vi "Create New Test Case.vi"(8 "error in (no error)":errorcluster, 10 "Path":path, 11 "Application":refnum<vi>) -> (0 "error out":errorcluster)   [LabVIEW 2020]
uses:
  <vilib>/LabVIEW Icon API/lv_icon/classes/Icon/Icon.lvclass
  <vilib>/LabVIEW Icon API/API_Rectangle Dimension.ctl
  <vilib>/LabVIEW Icon API/API_Text.ctl
  <vilib>/LabVIEW Icon API/API_Rectangle Colors.ctl
  <vilib>/Utility/sysdir.llb/System Directory Type.ctl
  <vilib>/Utility/error.llb/Error Cluster From Error Code.vi
  <vilib>/ErrorRing/Error Ring.xnode
  <vilib>/LabVIEW Icon API/LabVIEW Icon API.lvlib
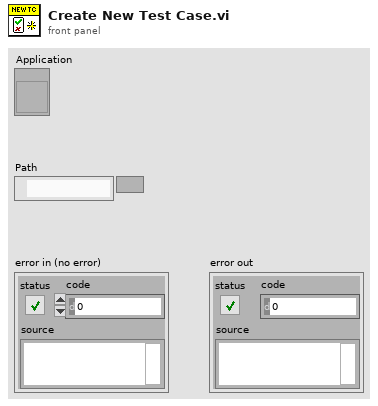
[diagram p1: front panel]
types:
  T1 = typedef "LabVIEW Icon API.lvlib/API_Rectangle Colors.ctl" = cluster{"Border":u32, "Background":u32}
  T2 = typedef "LabVIEW Icon API.lvlib/API_Text.ctl" = cluster{"Line 1 text":string, "Line 2 text":string, "Line 3 text":string, "Line 4 text":string}
  T3 = typedef "LabVIEW Icon API.lvlib/API_Rectangle Dimension.ctl" = cluster{"Width":i16, "Height":i16}
  T4 = typedef "System Directory Type.ctl" = i32
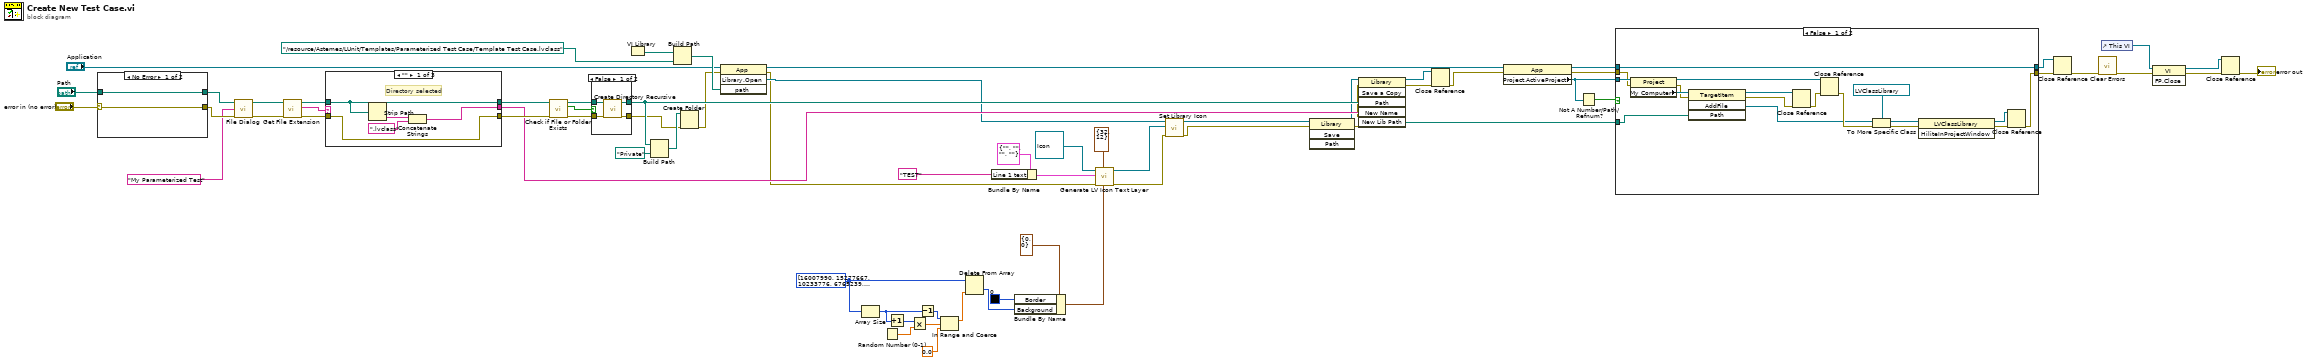
[diagram p0: block diagram]
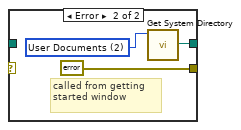
[diagram p2: hidden frame]
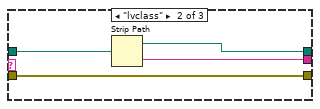
[diagram p3: hidden frame]
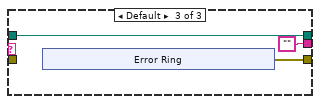
[diagram p4: hidden frame]
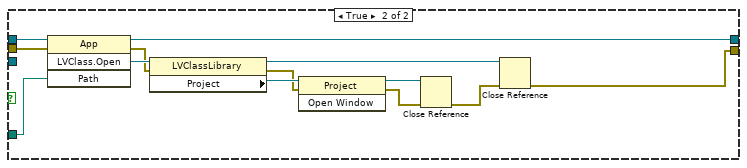
[diagram p6: hidden frame]
diagram:
  w12 = u32[] [16007990, 15277667, 10233776, 6765239, 4149685, 2201331, 240116, 48340, 38536, 5025616, 9159498, 13491257, 16771899, 16761095, 16750592, 16733986, 7951688, 10395294, 6323595] ("Array")
  n1 = case shown="No Error" "error in (no error)" {
    selector: "error in (no error)" -> [w69 _]
    tunnel: [w69 errorcluster {"status"=FALSE, "code"=0, "source"=""} ("error IO")] -> w38
    tunnel: [w68 w70] -> w39
    tunnel: "Path" -> [w68 _]
    frame No Error {
    }
    frame Error {
      w71 = T4 2 items=["User Home"=0, "User Desktop"=1, "User Documents"=2, "User Application Data"=3, "User Preferences"=4, "User Temporary"=5, "Public Documents"=6, "Public Application Data"=7, "Public Preferences"=8, "Public Cache"=13, "System Core Libraries"=9, "System Installed Libraries"=10, "Application Files"=11, "Boot Volume Root"=12] ("system directory type")
      # "called from getting started window"
      n2 = call <vilib>:"Get System Directory.vi"("system directory type"=w71) -> ("system directory"=w70:path)  [unwired: 10 in]
    }
  }
  n3 = call "File Dialog"("start path"=w39, "default name"="My Parameterized Test", "error in"=w38) -> ("selected path"=w64:path, "error out"=w37:errorcluster)  [unwired: 9 in, 2 out]
  n4 = call <vilib>:"Get File Extension.vi"("error in (no error)"=w37, "file"=w64) -> ("error out"=w67:errorcluster, "lowercase file extension"=w66:string, "dup file"=w65:path)  [unwired: 5 in, 2 out]
  n5 = case shown="\"\"" w66 {
    tunnel: w67 -> [w73 w78 _]
    tunnel: w65 -> [w74 w81 w82]
    tunnel: [w73 w78 w84] -> w62
    tunnel: [w75 w80 "" ("name")] -> w58
    tunnel: [w74 w79 w82] -> w63
    frame "" {
      # "Directory selected"
      n6 = Strip Path(path=w74) -> (name=w77:string)  [unwired: 1 out]
      n7 = Concatenate Strings(w77, ".lvclass" ("string")) -> (w75:string)
    }
    frame "lvclass" {
      n8 = Strip Path(path=w81) -> (stripped path=w79:path, name=w80:string)
    }
    frame Default {
      n9 = xnode "Error Ring"() -> ("error out"=w84:errorcluster)
    }
  }
  n10 = call <vilib>:"Check if File or Folder Exists.vi"("error in (no error)"=w62, "path"=w63) -> ("error out"=w61:errorcluster, "file or folder exists?"=w59:bool, "dup path"=w60:path)  [unwired: 7 in]
  n11 = case shown="False" w59 {
    tunnel: w61 -> [w92 w93]
    tunnel: w60 -> [w91 w94]
    tunnel: [w90 w94] -> w31
    tunnel: [w89 w93] -> w30
    frame False {
      n12 = call <vilib>:"Create Directory Recursive.vi"("error in (no error)"=w92, "directory"=w91) -> ("error out"=w89:errorcluster, "directory copy"=w90:path)  [unwired: 3 in, 1 out]
    }
    frame True {
    }
  }
  n13 = VI Library() -> (path=w51:path)
  n14 = Build Path(base path=w31, name or relative path=path "Private") -> (appended path=w33:path)
  n15 = Build Path(base path=w51, name or relative path=path "../resource/Astemes/LUnit/Templates/Parameterized Test Case/Template Test Case.lvclass") -> (appended path=w49:path)
  n16 = Create Folder(path (use dialog)=w33, error in=w30) -> (error out=w29:errorcluster)  [unwired: 1 in, 2 out]
  n17 = invoke class="App" method="Library.Open"(reference="Application", error in=w29, "path"=w49) -> (reference out=w26:refnum<vi>, error out=w22:errorcluster, "Open Library"=w25:refnum<vi>)  [unwired: 1 in, 1 out]
  n18 = Array Size(array=w12) -> (size(s)=w18:i32)
  n19 = Random Number (0-1)() -> (number: 0 to 1=w19:dbl)
  n20 = Increment(x=w18) -> (x+1=w17:i32)
  n21 = Multiply(x=w17, y=w19) -> (x*y=w14:dbl)
  n22 = Decrement(x=w18) -> (x-1=w15:i32)
  n23 = In Range and Coerce(upper limit=w15, x=w14, lower limit=0.0) -> (coerced(x)=w20:dbl)  [unwired: 1 out]
  n24 = Delete From Array(array=w12, index=w20) -> (deleted portion=w13:u32)  [unwired: 1 in, 1 out]
  n25 = Bundle By Name(cluster=T2 {"Line 1 text"="", "Line 2 text"="", "Line 3 text"="", "Line 4 text"=""} ("Text"), "Line 1 text"="TEST" ("Overlay Text")) -> (w6:T2)
  n26 = Bundle By Name(cluster=T1 {"Border"=0, "Background"=0} ("Library Color"), "Border"=u32 0 ("Background"), "Background"=w13) -> (w11:T1)
  n27 = call <vilib>:"Generate LV Icon Text Layer.vi"("Rectangle colors (black, white)"=w11, "Rectangle dimension (32,32)"=T3 {"Width"=32, "Height"=12}, "error in (no error)"=w22, "Text"=w6, "Icon in"=refnum<class "Icon.lvclass"> refnum ("Icon.lvclass in")) -> ("error out"=w8:errorcluster, "Icon out"=w5:refnum<class "Icon.lvclass">)  [unwired: 5 in]
  n28 = call <vilib>:"Set Library Icon.vi"("error in (no error)"=w8, "Icon"=w5, "Library Refnum in"=w25) -> ("error out"=w1:errorcluster, "Library Refnum out"=w21:refnum<vi>)  [unwired: 7 in]
  n29 = invoke class="Library" method="Save"(reference=w21, error in=w1) -> (reference out=w24:refnum<vi>, error out=w23:errorcluster)  [unwired: 2 in, 2 out]
  n30 = invoke class="Library" method="Save a Copy"(reference=w24, error in=w23, "Path"=w31, "New Name"=w58) -> (reference out=w47:refnum<vi>, error out=w46:errorcluster, "New Lib Path"=w28:path)  [unwired: 2 in, 3 out]
  n31 = Close Reference(reference=w47, error in (no error)=w46) -> (error out=w27:errorcluster)
  n32 = property class="App"(reference=w26, error in=w27) -> (reference out=w54:refnum<vi>, error out=w55:errorcluster, "Project.ActiveProject"=w56:refnum<vi>)
  n33 = Not A Number/Path/Refnum?(number/path/refnum=w56) -> (NaN/Path/Refnum?=w57:bool)
  n34 = case shown="False" w57 {
    tunnel: w56 -> [w112 _]
    tunnel: w55 -> [w110 w116]
    tunnel: w28 -> [w104 w114]
    tunnel: [w99 w113] -> w52
    tunnel: w54 -> [w103 w117]
    tunnel: [w103 w115] -> w53
    frame False {
      n35 = property class="Project"(reference=w112, error in=w110) -> (reference out=w106:refnum<vi>, error out=w109:errorcluster, "My Computer"=w111:refnum<vi>)
      n36 = invoke class="TargetItem" method="AddFile"(reference=w111, error in=w109, "Path"=w104) -> (reference out=w107:refnum<vi>, error out=w108:errorcluster, "AddFile"=w95:refnum<vi>)  [unwired: 1 in, 1 out]
      n37 = Close Reference(reference=w107, error in (no error)=w108) -> (error out=w105:errorcluster)
      n38 = Close Reference(reference=w106, error in (no error)=w105) -> (error out=w102:errorcluster)
      n39 = To More Specific Class(target class=refnum<vi> refnum ("reference"), reference=w95, error in=w102) -> (specific class reference=w96:refnum<vi>, error out=w98:errorcluster)
      n40 = invoke class="LVClassLibrary" method="HiliteInProjectWindow"(reference=w96, error in=w98) -> (reference out=w100:refnum<vi>, error out=w101:errorcluster)  [unwired: 1 in, 1 out]
      n41 = Close Reference(reference=w100, error in (no error)=w101) -> (error out=w99:errorcluster)
    }
    frame True {
      n42 = invoke class="App" method="LVClass.Open"(reference=w117, error in=w116, "Path"=w114) -> (reference out=w115:refnum<vi>, error out=w124:errorcluster, "LVClass.Open"=w125:refnum<vi>)  [unwired: 1 in, 1 out]
      n43 = property class="LVClassLibrary"(reference=w125, error in=w124) -> (reference out=w123:refnum<vi>, error out=w121:errorcluster, "Project"=w122:refnum<vi>)
      n44 = invoke class="Project" method="Open Window"(reference=w122, error in=w121) -> (reference out=w120:refnum<vi>, error out=w119:errorcluster)  [unwired: 1 in, 1 out]
      n45 = Close Reference(reference=w120, error in (no error)=w119) -> (error out=w118:errorcluster)
      n46 = Close Reference(reference=w123, error in (no error)=w118) -> (error out=w113:errorcluster)
    }
  }
  n47 = Close Reference(reference=w53, error in (no error)=w52) -> (error out=w48:errorcluster)
  n48 = call <vilib>:"Clear Errors.vi"("error in (no error)"=w48) -> ("error out"=w41:errorcluster)  [unwired: 5 in, 1 out]
  n49 = control-ref of="This VI"() -> (w45:refnum<vi>)
  n50 = invoke class="VI" method="FP.Close"(reference=w45, error in=w41) -> (reference out=w43:refnum<vi>, error out=w42:errorcluster)  [unwired: 1 in, 1 out]
  n51 = Close Reference(reference=w43, error in (no error)=w42) -> (error out=→"error out":errorcluster)
